vi "ConstructorString.vi"(6 "error in":errorcluster, 9 "DiagramDisable in":refnum<class "DiagramDisable.lvclass">) -> (0 "error out":errorcluster, 3 "DiagramDisable out":refnum<class "DiagramDisable.lvclass">, 4 "constructor":string)   [LabVIEW 2014, in "DiagramDisable.lvclass"]
uses:
  DiagramDisable.lvclass
  Structure/Structure.lvclass
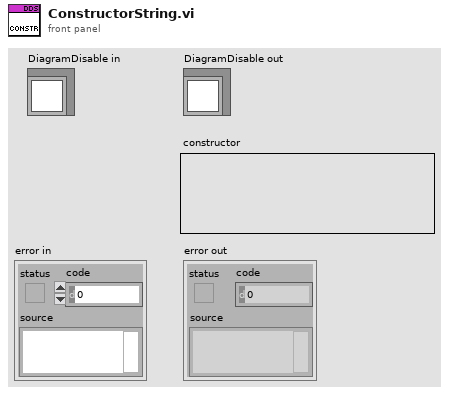
[diagram p1: front panel]
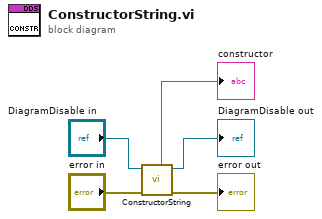
[diagram p0: block diagram]
diagram:
  n1 = call-parent "ConstructorString.vi"("error in"="error in", "Structure in"="DiagramDisable in") -> ("error out"=→"error out":errorcluster, "Structure out"=→"DiagramDisable out":refnum<class "DiagramDisable.lvclass">, "constructor"=→"constructor":string)  [unwired: 5 in]
